vi "Encoder Values.vi"(9 "Wheel Diameter":dbl=4.0, 10 "Encoder Position":dbl) -> (0 "Distance":dbl, 1 "Revolutions":dbl, 2 "Current Angle":dbl)   [LabVIEW 2018]
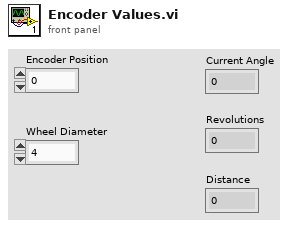
[diagram p1: front panel]
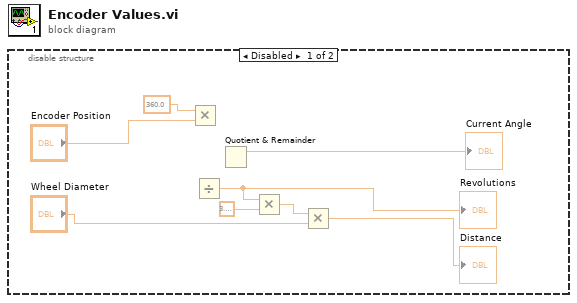
[diagram p0: block diagram]
diagram:
  n1 = disable-structure shown="Disabled" {
    frame Disabled {
      n2 = Multiply(x=360.0 ("y"), y="Encoder Position") -> ()  [unwired: 1 out]
      n3 = Divide() -> (x/y=w6:dbl)  [unwired: 2 in]
      "Revolutions" <- w6
      n4 = Quotient & Remainder() -> (x-y*floor(x/y)=→"Current Angle":dbl)  [unwired: 2 in, 1 out]
      n5 = Multiply(x=w6, y=3.141592653589793) -> (x*y=w7:dbl)
      n6 = Multiply(x=w7, y="Wheel Diameter") -> (x*y=→"Distance":dbl)
    }
    frame Enabled {
    }
  }
